vi "raised cosine fir.vi"(4 "data":fxp<+/-,16,1>=0.999969482421875) -> (1 "filtered":fxp<+/-,19,2>)   [LabVIEW 2014]
uses:
  <vilib>/rvi/FXPMathLib/basic elements/FxpDiscreteDelay/XNode/nifxpmath_DiscreteDelay.xnode
  <vilib>/rvi/FXPMathLib/FxpMul/XNode/nifxpmath_Multiplier.xnode
  <vilib>/rvi/FXPMathLib/FxpAdd/XNode/nifxpmath_Add.xnode
  <vilib>/rvi/FXPMathLib/sim/FxpSim.dll
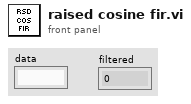
[diagram p1: front panel]
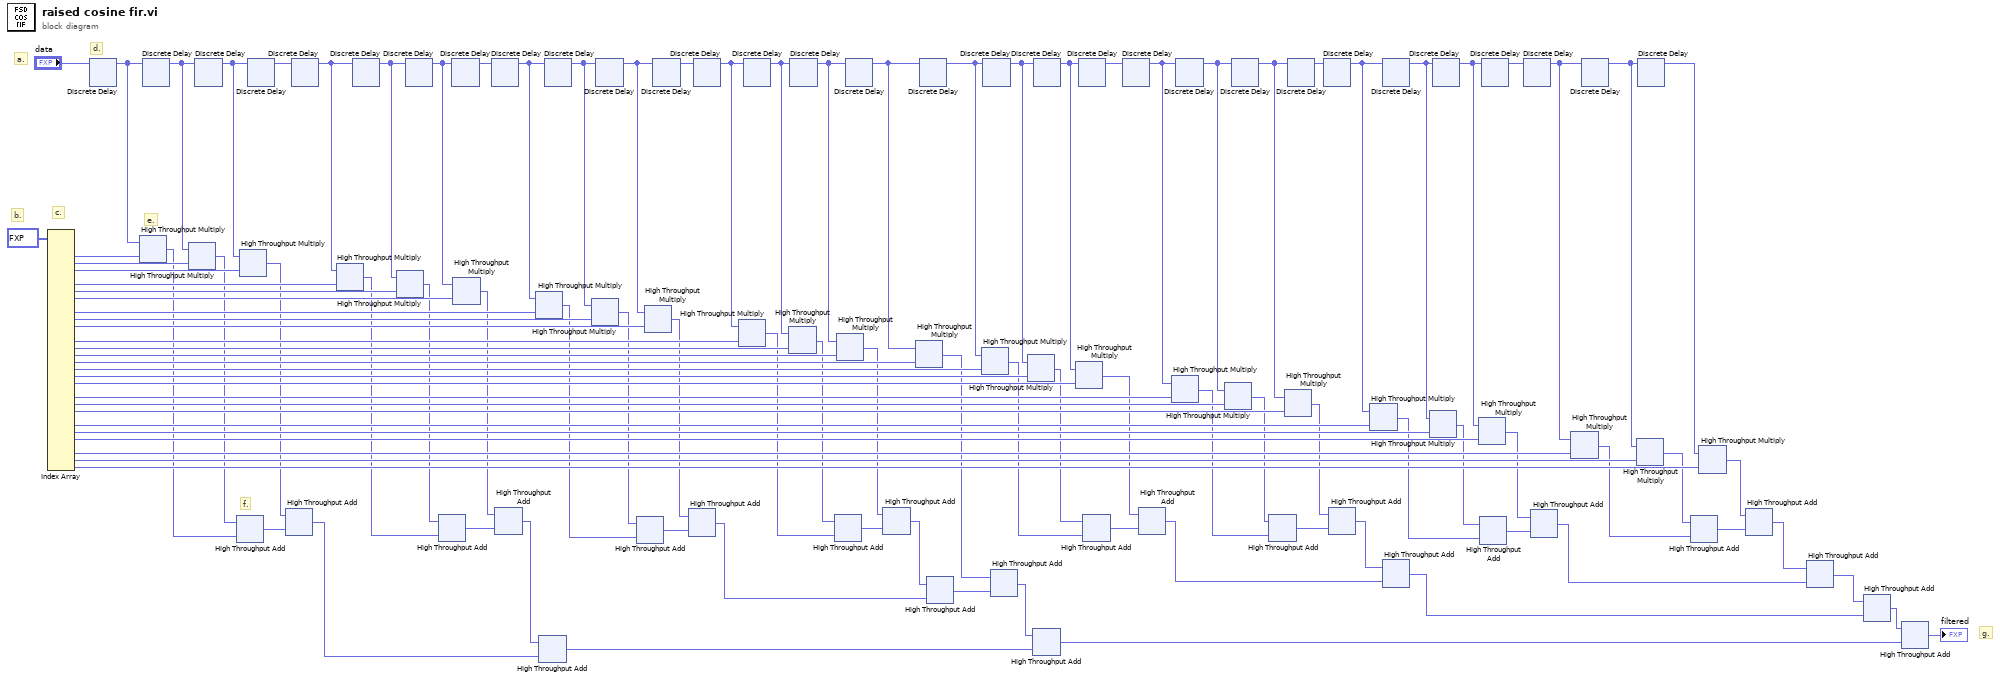
[diagram p0: block diagram]
diagram:
  # "g."
  # "f."
  # "e."
  # "d."
  # "c."
  # "b."
  # "a."
  n1 = Index Array(array=fxp<+/-,18,2>[] [0.0, 0.004241943359375, 0.0057220458984375, 0.002777099609375, 0.0, 0.0047760009765625, 0.01715087890625, 0.0227508544921875, 0.0, -0.0576171875, -0.1200408935546875, -0.12249755859375, 0.0, 0.2624969482421875, 0.6002044677734375, 0.887237548828125, 1.0, 0.887237548828125, 0.6002044677734375, 0.2624969482421875, 0.0, -0.12249755859375, -0.1200408935546875, -0.0576171875, 0.0, 0.0227508544921875, 0.01715087890625, 0.0047760009765625, 0.0, 0.002777099609375, 0.0057220458984375, 0.004241943359375, 0.0] ("Array")) -> (element #2=w2:fxp<+/-,18,2>, element #3=w106:fxp<+/-,18,2>, element #4=w105:fxp<+/-,18,2>, element #6=w104:fxp<+/-,18,2>, element #7=w103:fxp<+/-,18,2>, element #8=w102:fxp<+/-,18,2>, element #10=w101:fxp<+/-,18,2>, element #11=w100:fxp<+/-,18,2>, element #12=w99:fxp<+/-,18,2>, element #14=w98:fxp<+/-,18,2>, element #15=w97:fxp<+/-,18,2>, element #16=w96:fxp<+/-,18,2>, element #17=w95:fxp<+/-,18,2>, element #18=w94:fxp<+/-,18,2>, element #19=w93:fxp<+/-,18,2>, element #20=w92:fxp<+/-,18,2>, element #22=w91:fxp<+/-,18,2>, element #23=w90:fxp<+/-,18,2>, element #24=w89:fxp<+/-,18,2>, element #26=w88:fxp<+/-,18,2>, element #27=w87:fxp<+/-,18,2>, element #28=w86:fxp<+/-,18,2>, element #30=w85:fxp<+/-,18,2>, element #31=w84:fxp<+/-,18,2>, element #32=w83:fxp<+/-,18,2>)  [unwired: 32 in, 7 out]
  n2 = xnode ("Discrete Delay")("D"="data") -> ("Q"=w3:fxp<+/-,16,1>)
  n3 = xnode ("High Throughput Multiply")("x"=w3, "y"=w2) -> ("x*y"=w81:fxp<+/-,19,2>)
  n4 = xnode ("Discrete Delay")("D"=w3) -> ("Q"=w33:fxp<+/-,16,1>)
  n5 = xnode ("High Throughput Multiply")("x"=w33, "y"=w106) -> ("x*y"=w82:fxp<+/-,19,2>)
  n6 = xnode ("Discrete Delay")("D"=w33) -> ("Q"=w32:fxp<+/-,16,1>)
  n7 = xnode ("High Throughput Add")("x"=w82, "y"=w81) -> ("x+y"=w79:fxp<+/-,19,2>)
  n8 = xnode ("High Throughput Multiply")("x"=w32, "y"=w105) -> ("x*y"=w80:fxp<+/-,19,2>)
  n9 = xnode ("Discrete Delay")("D"=w32) -> ("Q"=w31:fxp<+/-,16,1>)
  n10 = xnode ("High Throughput Add")("x"=w80, "y"=w79) -> ("x+y"=w73:fxp<+/-,19,2>)
  n11 = xnode ("Discrete Delay")("D"=w31) -> ("Q"=w30:fxp<+/-,16,1>)
  n12 = xnode ("High Throughput Multiply")("x"=w30, "y"=w104) -> ("x*y"=w77:fxp<+/-,19,2>)
  n13 = xnode ("Discrete Delay")("D"=w30) -> ("Q"=w29:fxp<+/-,16,1>)
  n14 = xnode ("High Throughput Multiply")("x"=w29, "y"=w103) -> ("x*y"=w78:fxp<+/-,19,2>)
  n15 = xnode ("Discrete Delay")("D"=w29) -> ("Q"=w28:fxp<+/-,16,1>)
  n16 = xnode ("High Throughput Add")("x"=w78, "y"=w77) -> ("x+y"=w75:fxp<+/-,19,2>)
  n17 = xnode ("Discrete Delay")("D"=w28) -> ("Q"=w27:fxp<+/-,16,1>)
  n18 = xnode ("High Throughput Multiply")("x"=w28, "y"=w102) -> ("x*y"=w76:fxp<+/-,19,2>)
  n19 = xnode ("Discrete Delay")("D"=w27) -> ("Q"=w26:fxp<+/-,16,1>)
  n20 = xnode ("High Throughput Add")("x"=w76, "y"=w75) -> ("x+y"=w74:fxp<+/-,19,2>)
  n21 = xnode ("High Throughput Multiply")("x"=w26, "y"=w101) -> ("x*y"=w71:fxp<+/-,19,2>)
  n22 = xnode ("High Throughput Add")("x"=w74, "y"=w73) -> ("x+y"=w59:fxp<+/-,19,2>)
  n23 = xnode ("Discrete Delay")("D"=w26) -> ("Q"=w25:fxp<+/-,16,1>)
  n24 = xnode ("High Throughput Multiply")("x"=w25, "y"=w100) -> ("x*y"=w72:fxp<+/-,19,2>)
  n25 = xnode ("Discrete Delay")("D"=w25) -> ("Q"=w24:fxp<+/-,16,1>)
  n26 = xnode ("High Throughput Add")("x"=w72, "y"=w71) -> ("x+y"=w69:fxp<+/-,19,2>)
  n27 = xnode ("High Throughput Multiply")("x"=w24, "y"=w99) -> ("x*y"=w70:fxp<+/-,19,2>)
  n28 = xnode ("Discrete Delay")("D"=w24) -> ("Q"=w23:fxp<+/-,16,1>)
  n29 = xnode ("High Throughput Add")("x"=w70, "y"=w69) -> ("x+y"=w63:fxp<+/-,19,2>)
  n30 = xnode ("Discrete Delay")("D"=w23) -> ("Q"=w22:fxp<+/-,16,1>)
  n31 = xnode ("High Throughput Multiply")("x"=w22, "y"=w98) -> ("x*y"=w67:fxp<+/-,19,2>)
  n32 = xnode ("Discrete Delay")("D"=w22) -> ("Q"=w21:fxp<+/-,16,1>)
  n33 = xnode ("High Throughput Multiply")("x"=w21, "y"=w97) -> ("x*y"=w68:fxp<+/-,19,2>)
  n34 = xnode ("Discrete Delay")("D"=w21) -> ("Q"=w20:fxp<+/-,16,1>)
  n35 = xnode ("High Throughput Add")("x"=w68, "y"=w67) -> ("x+y"=w65:fxp<+/-,19,2>)
  n36 = xnode ("High Throughput Multiply")("x"=w20, "y"=w96) -> ("x*y"=w66:fxp<+/-,19,2>)
  n37 = xnode ("Discrete Delay")("D"=w20) -> ("Q"=w19:fxp<+/-,16,1>)
  n38 = xnode ("High Throughput Add")("x"=w66, "y"=w65) -> ("x+y"=w64:fxp<+/-,19,2>)
  n39 = xnode ("High Throughput Multiply")("x"=w19, "y"=w95) -> ("x*y"=w62:fxp<+/-,19,2>)
  n40 = xnode ("Discrete Delay")("D"=w19) -> ("Q"=w18:fxp<+/-,16,1>)
  n41 = xnode ("High Throughput Add")("x"=w64, "y"=w63) -> ("x+y"=w61:fxp<+/-,19,2>)
  n42 = xnode ("High Throughput Multiply")("x"=w18, "y"=w94) -> ("x*y"=w57:fxp<+/-,19,2>)
  n43 = xnode ("Discrete Delay")("D"=w18) -> ("Q"=w17:fxp<+/-,16,1>)
  n44 = xnode ("High Throughput Add")("x"=w62, "y"=w61) -> ("x+y"=w60:fxp<+/-,19,2>)
  n45 = xnode ("High Throughput Multiply")("x"=w17, "y"=w93) -> ("x*y"=w58:fxp<+/-,19,2>)
  n46 = xnode ("High Throughput Add")("x"=w60, "y"=w59) -> ("x+y"=w35:fxp<+/-,19,2>)
  n47 = xnode ("Discrete Delay")("D"=w17) -> ("Q"=w16:fxp<+/-,16,1>)
  n48 = xnode ("High Throughput Multiply")("x"=w16, "y"=w92) -> ("x*y"=w56:fxp<+/-,19,2>)
  n49 = xnode ("Discrete Delay")("D"=w16) -> ("Q"=w15:fxp<+/-,16,1>)
  n50 = xnode ("High Throughput Add")("x"=w58, "y"=w57) -> ("x+y"=w55:fxp<+/-,19,2>)
  n51 = xnode ("Discrete Delay")("D"=w15) -> ("Q"=w14:fxp<+/-,16,1>)
  n52 = xnode ("High Throughput Add")("x"=w56, "y"=w55) -> ("x+y"=w49:fxp<+/-,19,2>)
  n53 = xnode ("High Throughput Multiply")("x"=w14, "y"=w91) -> ("x*y"=w53:fxp<+/-,19,2>)
  n54 = xnode ("Discrete Delay")("D"=w14) -> ("Q"=w13:fxp<+/-,16,1>)
  n55 = xnode ("High Throughput Multiply")("x"=w13, "y"=w90) -> ("x*y"=w54:fxp<+/-,19,2>)
  n56 = xnode ("Discrete Delay")("D"=w13) -> ("Q"=w12:fxp<+/-,16,1>)
  n57 = xnode ("High Throughput Add")("x"=w54, "y"=w53) -> ("x+y"=w51:fxp<+/-,19,2>)
  n58 = xnode ("High Throughput Multiply")("x"=w12, "y"=w89) -> ("x*y"=w52:fxp<+/-,19,2>)
  n59 = xnode ("Discrete Delay")("D"=w12) -> ("Q"=w11:fxp<+/-,16,1>)
  n60 = xnode ("Discrete Delay")("D"=w11) -> ("Q"=w1:fxp<+/-,16,1>)
  n61 = xnode ("High Throughput Add")("x"=w52, "y"=w51) -> ("x+y"=w50:fxp<+/-,19,2>)
  n62 = xnode ("High Throughput Multiply")("x"=w1, "y"=w88) -> ("x*y"=w47:fxp<+/-,19,2>)
  n63 = xnode ("Discrete Delay")("D"=w1) -> ("Q"=w10:fxp<+/-,16,1>)
  n64 = xnode ("High Throughput Add")("x"=w50, "y"=w49) -> ("x+y"=w37:fxp<+/-,19,2>)
  n65 = xnode ("High Throughput Multiply")("x"=w10, "y"=w87) -> ("x*y"=w48:fxp<+/-,19,2>)
  n66 = xnode ("Discrete Delay")("D"=w10) -> ("Q"=w9:fxp<+/-,16,1>)
  n67 = xnode ("High Throughput Multiply")("x"=w9, "y"=w86) -> ("x*y"=w46:fxp<+/-,19,2>)
  n68 = xnode ("High Throughput Add")("x"=w48, "y"=w47) -> ("x+y"=w45:fxp<+/-,19,2>)
  n69 = xnode ("Discrete Delay")("D"=w9) -> ("Q"=w8:fxp<+/-,16,1>)
  n70 = xnode ("Discrete Delay")("D"=w8) -> ("Q"=w7:fxp<+/-,16,1>)
  n71 = xnode ("High Throughput Add")("x"=w46, "y"=w45) -> ("x+y"=w39:fxp<+/-,19,2>)
  n72 = xnode ("High Throughput Multiply")("x"=w7, "y"=w85) -> ("x*y"=w43:fxp<+/-,19,2>)
  n73 = xnode ("Discrete Delay")("D"=w7) -> ("Q"=w6:fxp<+/-,16,1>)
  n74 = xnode ("High Throughput Multiply")("x"=w6, "y"=w84) -> ("x*y"=w44:fxp<+/-,19,2>)
  n75 = xnode ("Discrete Delay")("D"=w6) -> ("Q"=w5:fxp<+/-,16,1>)
  n76 = xnode ("High Throughput Add")("x"=w44, "y"=w43) -> ("x+y"=w41:fxp<+/-,19,2>)
  n77 = xnode ("High Throughput Multiply")("x"=w5, "y"=w83) -> ("x*y"=w42:fxp<+/-,19,2>)
  n78 = xnode ("High Throughput Add")("x"=w42, "y"=w41) -> ("x+y"=w40:fxp<+/-,19,2>)
  n79 = xnode ("High Throughput Add")("x"=w40, "y"=w39) -> ("x+y"=w38:fxp<+/-,19,2>)
  n80 = xnode ("High Throughput Add")("x"=w38, "y"=w37) -> ("x+y"=w36:fxp<+/-,19,2>)
  n81 = xnode ("High Throughput Add")("x"=w36, "y"=w35) -> ("x+y"=→"filtered":fxp<+/-,19,2>)
